vi "PV Handheld Gauge Data.vi"(8 "error in (no error)":errorcluster, 9 "Handheld Gauge Data-Cluster":T1={"Parameter"=0, "Parameter\nread only<->describe"=FALSE, "Correction facktor\n(0,20 - 8,00) "=1.0, "Physical units"=0} {"Physical units" items=["mbar", "Pa", "Atm", "Torr", "hPa "]; "Correction facktor\n(0,20 - 8,00)" min=0.2 max=8 step=0.01 format="%.2f"; "Parameter" items=[" Pressure (read only) [mbar]", " Correction factor Pirani", " Actual error code (read only)", " Software version Transmitter  (read only)", " Unit type Transmitter (read only)", " Physical units"]}, 10 "Adress of unit":u16=1 max=999 step=1, 11 "VISA session":refnum<visa-resource-name>) -> (0 "error out":errorcluster, 2 "response (data)":string, 3 "dup VISA session":refnum<visa-resource-name>)   [LabVIEW 2021, in "Pfeiffer Vacuum.lvlib"]
doc: "There are 6 parameters available, only one of which can be enabled at a time. \n\n0 - Pressure (read only) [mbar] (default)\n1 - Correction factor Pirani \n2 - Actual error code (read only)\n3 - Software version Transmitter (read only)\n4 - Unit type Transmitter (read only)\n5 - Physical units \n\nNote: The 6 controls right of this one will set the appropriate values for the selected parameter. Any settings for an parameter that is not selected will be ignored. If a value is out of range, it will be changed to either the upper or the lower limit of the range."
uses:
  <instrlib>/Pfeiffer Vacuum/Pfeiffer Vacuum.lvlib
  <instrlib>/Pfeiffer Vacuum/Public/Handheld Gauge/PV Handheld Gauge Data - Cluster.ctl
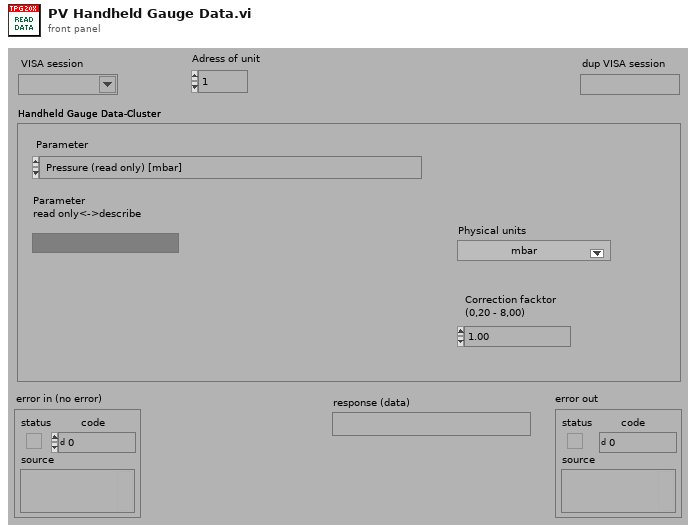
[diagram p1: front panel]
types:
  T1 = typedef "Pfeiffer Vacuum.lvlib/PV Handheld Gauge Data - Cluster.ctl" = cluster{"Parameter":u16, "Parameter\nread only<->describe":bool, "Correction facktor\n(0,20 - 8,00) ":sgl, "Physical units":u16}
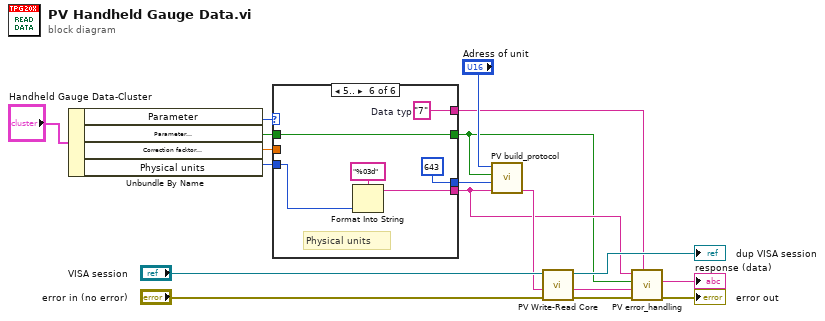
[diagram p0: block diagram]
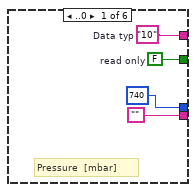
[diagram p2: hidden frame]
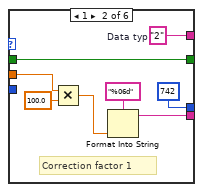
[diagram p3: hidden frame]
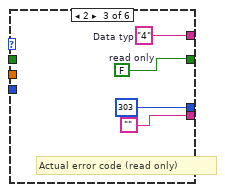
[diagram p4: hidden frame]
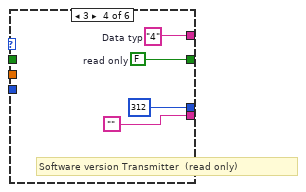
[diagram p5: hidden frame]
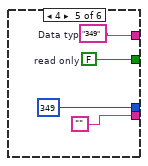
[diagram p6: hidden frame]
diagram:
  n1 = Unbundle By Name("Handheld Gauge Data-Cluster") -> ("Parameter"=w16:u16, "Parameter\nread only<->describe"=w15:bool, "Correction facktor\n(0,20 - 8,00)"=w3:sgl, "Physical units"=w2:u16)
  n2 = case shown="5.." w16 {
    tunnel: [u16 740 ("Parameter-number") u16 742 ("Parameter-number") u16 303 ("Parameter-number") u16 312 ("Parameter-number") u16 349 ("Parameter-number") u16 643 ("Parameter-number")] -> w17
    tunnel: ["" w24 "" "" "" w43] -> w6
    tunnel: [w20 w29 w33 w36 w42 w47] -> w5
    tunnel: w15 -> [_ w29 _ _ _ w47]
    tunnel: [w21 w28 w31 w35 w39 w46] -> w7
    tunnel: w3 -> [_ w23 _ _ _ _]
    tunnel: w2 -> [_ _ _ _ _ w44]
    frame ..0 {
      w20 = FALSE  # read only
      w21 = "10"  # Data typ
      # "Pressure  [mbar]"
    }
    frame 1 {
      w28 = "2"  # Data typ
      # "Correction factor 1"
      n3 = Multiply(x=w23, y=100.0) -> (x*y=w25:dbl)
      n4 = Format Into String(format string="%06d" ("Format-String"), w25) -> (resulting string=w24:string)  [unwired: 2 in, 1 out]
    }
    frame 2 {
      w31 = "4"  # Data typ
      w33 = FALSE  # read only
      # "Actual error code (read only)"
    }
    frame 3 {
      w35 = "4"  # Data typ
      w36 = FALSE  # read only
      # "Software version Transmitter  (read only)"
    }
    frame 4 {
      w39 = "349"  # Data typ
      w42 = FALSE  # read only
    }
    frame 5.. {
      w46 = "7"  # Data typ
      # "Physical units"
      n5 = Format Into String(format string="%03d" ("Format-String"), w44) -> (resulting string=w43:string)  [unwired: 2 in, 1 out]
    }
  }
  n6 = call <instrlib>:"PV build_protocol.vi"("Data"=w6, "Parameter-number"=w17, "parameter\nread<->describe"=w5, "Adress"="Adress of unit") -> ("output"=w11:string)  [unwired: 3 in]
  n7 = call <instrlib>:"PV Write-Read Core.vi"("error in"="error in (no error)", "Write data in"=w11, "VISA session"="VISA session") -> ("error out"=w8:errorcluster, "response (data) out"=w9:string, "dup VISA session"=→"dup VISA session":refnum<visa-resource-name>)  [unwired: 2 in]
  n8 = call <instrlib>:"PV error_handling.vi"("Data Typ in"=w7, "error in"=w8, "response (data) in"=w9, "Parameter\nread only<->describe"=w5, "data in"=w6) -> ("error out"=→"error out":errorcluster, "Data out"=→"response (data)":string)  [unwired: 4 in, 1 out]
